vi "Playing.vi"() -> ()   [LabVIEW 2015]
uses:
  SubVIs/Module.Input.ctl
  SubVIs/Loop.Type.ctl
  SubVIs/Module.Type.ctl
  SubVIs/Input.Type.ctl
  SubVIs/Module.Output.ctl
  SubVIs/Output.Type.ctl
  Classes/Loop/Block Diagram/Block Diagram.lvclass
panel:
  out "error out":errorcluster
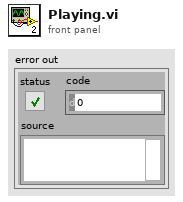
[diagram p1: front panel]
types:
  T1 = cluster{"Name":string, "Type":enum16{"DebugDMA", "Directional Memory", "Analog Replay Memory", "Pattern Generation Memory"}}
  T2 = typedef "Module.Input.ctl" = cluster{"Owning.Loop":T3, "Mod.Type":T4, "Mod.Name":string, "Channels":cluster{"IO Name":string, "Signal Name":string, "Type":T5}[]}
  T3 = typedef "Loop.Type.ctl" = enum16{"HighSpeedDigital", "LowSpeedSigital", "AnalogOutput", "AnalogInput"}
  T4 = typedef "Module.Type.ctl" = enum16{"Digital.8 Channels", "Digital.32 Channels", "Analog.16 Channels.FXP24.5"}
  T5 = typedef "Input.Type.ctl" = enum16{"Digital PWM Input", "Digital Static Input", "Analog PWM Input", "Digital Direct Input", "Analog Direct Input", "Digital Event"}
  T6 = enum16{"DebugDMA", "Directional Memory", "Analog Replay Memory", "Pattern Generation Memory"}
  T7 = typedef "Module.Output.ctl" = cluster{"Owning.Loop":T3, "Mod.Type":T4, "Mod.Name":string, "Channels":cluster{"IO Name":string, "Signal Name":string, "Type":T8}[]}
  T8 = typedef "Output.Type.ctl" = enum16{"Digital PWM Output", "Digital Static Output", "Analog Sine Output", "Digital Direct", "Analog Direct", "Analog Replay", "Pattern Generation", "Directional", "Analog Knock"}
  T9 = cluster{"Name":string, "Type":enum16{"DebugDMA", "Directional Memory", "Analog Replay Memory", "Pattern Generation Memory"}}[]
  T10 = cluster{"IO Name":string, "Signal Name":string, "Type":T8}[]
  T11 = typedef "Variables.ctl" = cluster{"Loops":cluster{"Digital.HighSpeed":cluster{"Diagram":refnum<vi>, "Tunnel":refnum<vi>}, "Digital.LowSpeed":cluster{"Diagram":refnum<vi>, "Tunnel":refnum<vi>}, "Analog.Output":cluster{"Diagram":refnum<vi>, "Tunnel":refnum<vi>}, "Analog.Input":cluster{"Diagram":refnum<vi>, "Tunnel":refnum<vi>}}, "DMA":refnum<vi>, "Locations":cluster{"Sequence.Init":refnum<vi>}, "Application Directory":path, "Block Diagram":refnum<vi>, "vi.Lib":path}
  T12 = typedef "LVPointTypeDef.ctl" = cluster{"Horizontal":i16, "Vertical":i16}
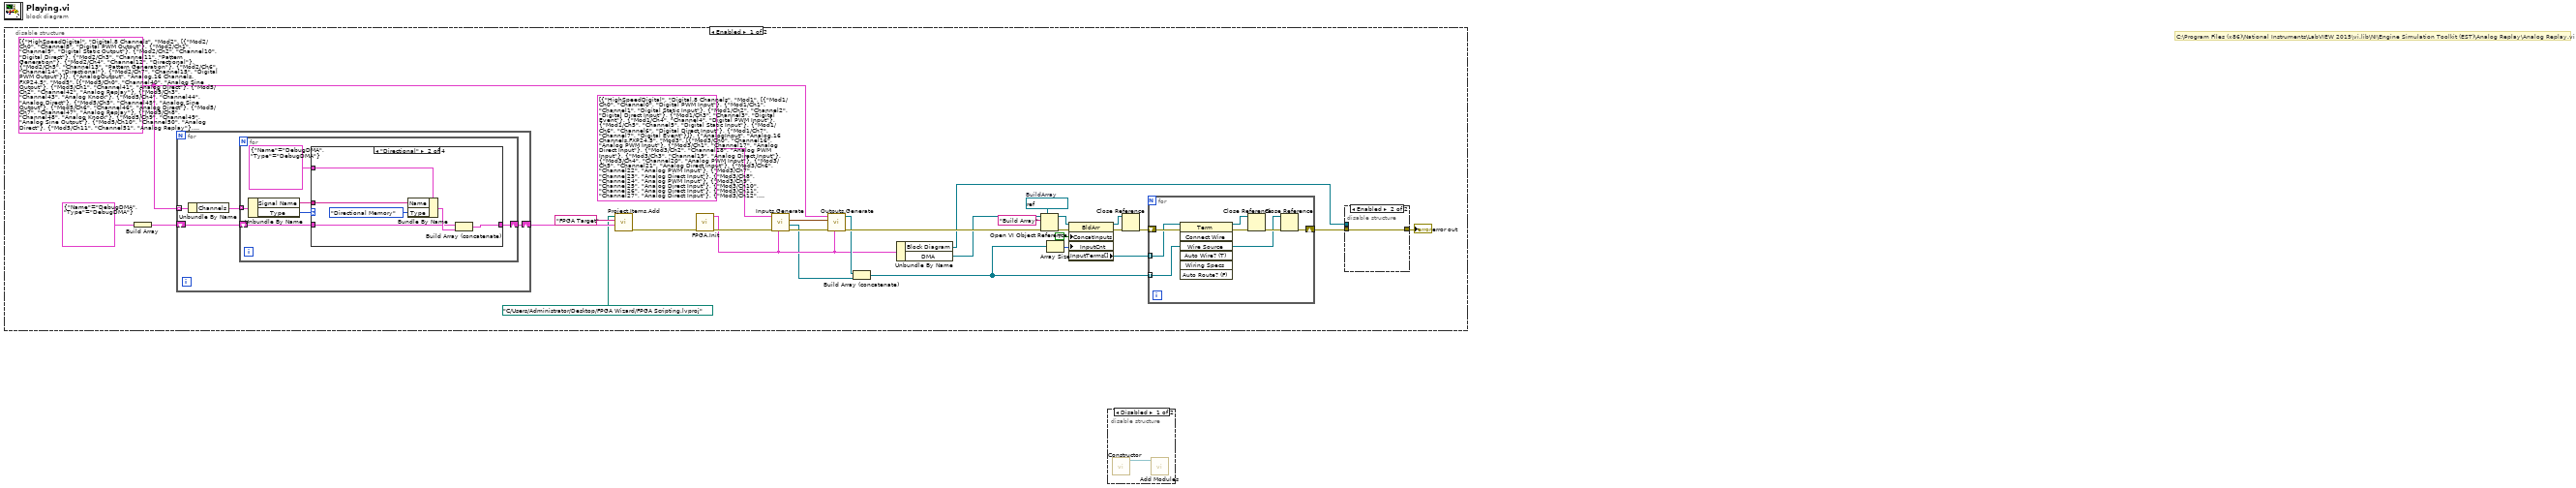
[diagram p0: block diagram]
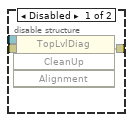
[diagram p3: hidden frame]
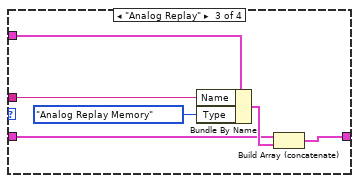
[diagram p5: hidden frame]
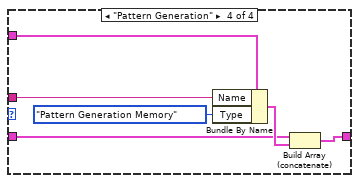
[diagram p6: hidden frame]
diagram:
  # "C:\\Program Files (x86)\\National Instruments\\LabVIEW 2015\\vi.lib\\NI\\Engine Simulation Toolkit (EST)\\Analog Replay\\Analog Replay.vi"
  n1 = disable-structure shown="Enabled" {
    frame Enabled {
      w11 = T7[] [{"Owning.Loop"=enum."HighSpeedDigital", "Mod.Type"=enum."Digital.8 Channels", "Mod.Name"="Mod2", "Channels"=[{"IO Name"="Mod2/Ch0", "Signal Name"="Channel8", "Type"=enum."Digital PWM Output"}, {"IO Name"="Mod2/Ch1", "Signal Name"="Channel9", "Type"=enum."Digital Static Output"}, {"IO Name"="Mod2/Ch2", "Signal Name"="Channel10", "Type"=enum."Digital Direct"}, {"IO Name"="Mod2/Ch3", "Signal Name"="Channel11", "Type"=enum."Pattern Generation"}, {"IO Name"="Mod2/Ch4", "Signal Name"="Channel12", "Type"=enum."Directional"}, {"IO Name"="Mod2/Ch5", "Signal Name"="Channel13", "Type"=enum."Pattern Generation"}, {"IO Name"="Mod2/Ch6", "Signal Name"="Channel14", "Type"=enum."Directional"}, {"IO Name"="Mod2/Ch7", "Signal Name"="Channel15", "Type"=enum."Digital PWM Output"}]}, {"Owning.Loop"=enum."AnalogOutput", "Mod.Type"=enum."Analog.16 Channels.FXP24.5", "Mod.Name"="Mod5", "Channels"=[{"IO Name"="Mod5/Ch0", "Signal Name"="Channel40", "Type"=enum."Analog Sine Output"}, {"IO Name"="Mod5/Ch1", "Signal Name"="Channel41", "Type"=enum."Analog Direct"}, {"IO Name"="Mod5/Ch2", "Signal Name"="Channel42", "Type"=enum."Analog Replay"}, {"IO Name"="Mod5/Ch3", "Signal Name"="Channel43", "Type"=enum."Analog Knock"}, {"IO Name"="Mod5/Ch4", "Signal Name"="Channel44", "Type"=enum."Analog Direct"}, {"IO Name"="Mod5/Ch5", "Signal Name"="Channel45", "Type"=enum."Analog Sine Output"}, {"IO Name"="Mod5/Ch6", "Signal Name"="Channel46", "Type"=enum."Analog Direct"}, {"IO Name"="Mod5/Ch7", "Signal Name"="Channel47", "Type"=enum."Analog Replay"}, {"IO Name"="Mod5/Ch8", "Signal Name"="Channel48", "Type"=enum."Analog Knock"}, {"IO Name"="Mod5/Ch9", "Signal Name"="Channel49", "Type"=enum."Analog Sine Output"}, {"IO Name"="Mod5/Ch10", "Signal Name"="Channel50", "Type"=enum."Analog Direct"}, {"IO Name"="Mod5/Ch11", "Signal Name"="Channel51", "Type"=enum."Analog Replay"}, {"IO Name"="Mod5/Ch12", "Signal Name"="Channel52", "Type"=enum."Analog Knock"}, {"IO Name"="Mod5/Ch13", "Signal Name"="Channel53", "Type"=enum."Analog Replay"}, {"IO Name"="Mod5/Ch14", "Signal Name"="Channel54", "Type"=enum."Analog Direct"}, {"IO Name"="Mod5/Ch15", "Signal Name"="Channel55", "Type"=enum."Analog Sine Output"}]}] ("Outputs")
      w29 = refnum<vi> refnum  # BuildArray
      n2 = Build Array(T1 {"Name"="DebugDMA", "Type"=enum."DebugDMA"}) -> (w9:T9)
      n3 = for {
        tunnel: w11 -> [w45] mode=indexing
        shift-right: [w42] -> w8
        shift-left: w9 -> [w43]
        n4 = Unbundle By Name(w45) -> ("Channels"=w44:T10)
        n5 = for {
          tunnel: w44 -> [w51] mode=indexing
          shift-right: [w46] -> w42
          shift-left: w43 -> [w47]
          n6 = Unbundle By Name(w51) -> ("Signal Name"=w49:string, "Type"=w50:T8)
          n7 = case shown="\"Directional\"" w50 {
            tunnel: w49 -> [_ w57 w63 w69]
            tunnel: T1 {"Name"="DebugDMA", "Type"=enum."DebugDMA"} -> [_ w58 w64 w70]
            tunnel: w47 -> [w52 w54 w60 w66]
            tunnel: [w52 w53 w59 w65] -> w46
            frame Default {
            }
            frame "Directional" {
              n8 = Bundle By Name(cluster=w58, "Name"=w57, "Type"=T6."Directional Memory") -> (w55:T1)
              n9 = Build Array (concatenate)(w54, w55) -> (w53:T9)
            }
            frame "Analog Replay" {
              n10 = Bundle By Name(cluster=w64, "Name"=w63, "Type"=T6."Analog Replay Memory") -> (w61:T1)
              n11 = Build Array (concatenate)(w60, w61) -> (w59:T9)
            }
            frame "Pattern Generation" {
              n12 = Bundle By Name(cluster=w70, "Name"=w69, "Type"=T6."Pattern Generation Memory") -> (w67:T1)
              n13 = Build Array (concatenate)(w66, w67) -> (w65:T9)
            }
          }
        }
      }
      n14 = call "Project.Items.Add.vi"("Array"=w8, "FPGA Target Name"="FPGA Target", "Path"=path "C:/Users/Administrator/Desktop/FPGA Wizard/FPGA Scripting.lvproj") -> ("error out"=w18:errorcluster)  [unwired: 8 in]
      n15 = call "FPGA.Init.vi"("error in (no error)"=w18) -> ("error out"=w19:errorcluster, "Cluster"=w5:T11)  [unwired: 9 in]
      n16 = call "Inputs.Generate.vi"("Variables"=w5, "error in (no error)"=w19, "Inputs"=T2[] [{"Owning.Loop"=enum."HighSpeedDigital", "Mod.Type"=enum."Digital.8 Channels", "Mod.Name"="Mod1", "Channels"=[{"IO Name"="Mod1/Ch0", "Signal Name"="Channel0", "Type"=enum."Digital PWM Input"}, {"IO Name"="Mod1/Ch1", "Signal Name"="Channel1", "Type"=enum."Digital Static Input"}, {"IO Name"="Mod1/Ch2", "Signal Name"="Channel2", "Type"=enum."Digital Direct Input"}, {"IO Name"="Mod1/Ch3", "Signal Name"="Channel3", "Type"=enum."Digital Event"}, {"IO Name"="Mod1/Ch4", "Signal Name"="Channel4", "Type"=enum."Digital PWM Input"}, {"IO Name"="Mod1/Ch5", "Signal Name"="Channel5", "Type"=enum."Digital Static Input"}, {"IO Name"="Mod1/Ch6", "Signal Name"="Channel6", "Type"=enum."Digital Direct Input"}, {"IO Name"="Mod1/Ch7", "Signal Name"="Channel7", "Type"=enum."Digital Event"}]}, {"Owning.Loop"=enum."AnalogInput", "Mod.Type"=enum."Analog.16 Channels.FXP24.5", "Mod.Name"="Mod3", "Channels"=[{"IO Name"="Mod3/Ch0", "Signal Name"="Channel16", "Type"=enum."Analog PWM Input"}, {"IO Name"="Mod3/Ch1", "Signal Name"="Channel17", "Type"=enum."Analog Direct Input"}, {"IO Name"="Mod3/Ch2", "Signal Name"="Channel18", "Type"=enum."Analog PWM Input"}, {"IO Name"="Mod3/Ch3", "Signal Name"="Channel19", "Type"=enum."Analog Direct Input"}, {"IO Name"="Mod3/Ch4", "Signal Name"="Channel20", "Type"=enum."Analog PWM Input"}, {"IO Name"="Mod3/Ch5", "Signal Name"="Channel21", "Type"=enum."Analog Direct Input"}, {"IO Name"="Mod3/Ch6", "Signal Name"="Channel22", "Type"=enum."Analog PWM Input"}, {"IO Name"="Mod3/Ch7", "Signal Name"="Channel23", "Type"=enum."Analog Direct Input"}, {"IO Name"="Mod3/Ch8", "Signal Name"="Channel24", "Type"=enum."Analog PWM Input"}, {"IO Name"="Mod3/Ch9", "Signal Name"="Channel25", "Type"=enum."Analog Direct Input"}, {"IO Name"="Mod3/Ch10", "Signal Name"="Channel26", "Type"=enum."Analog Direct Input"}, {"IO Name"="Mod3/Ch11", "Signal Name"="Channel27", "Type"=enum."Analog Direct Input"}, {"IO Name"="Mod3/Ch12", "Signal Name"="Channel28", "Type"=enum."Analog Direct Input"}, {"IO Name"="Mod3/Ch13", "Signal Name"="Channel29", "Type"=enum."Analog Direct Input"}, {"IO Name"="Mod3/Ch14", "Signal Name"="Channel30", "Type"=enum."Analog Direct Input"}, {"IO Name"="Mod3/Ch15", "Signal Name"="Channel31", "Type"=enum."Analog PWM Input"}]}, {"Owning.Loop"=enum."HighSpeedDigital", "Mod.Type"=enum."Digital.8 Channels", "Mod.Name"="Mod4", "Channels"=[{"IO Name"="Mod4/Ch0", "Signal Name"="Channel32", "Type"=enum."Digital PWM Input"}, {"IO Name"="Mod4/Ch1", "Signal Name"="Channel33", "Type"=enum."Digital Static Input"}, {"IO Name"="Mod4/Ch2", "Signal Name"="Channel34", "Type"=enum."Digital Direct Input"}, {"IO Name"="Mod4/Ch3", "Signal Name"="Channel35", "Type"=enum."Digital Event"}, {"IO Name"="Mod4/Ch4", "Signal Name"="Channel36", "Type"=enum."Digital PWM Input"}, {"IO Name"="Mod4/Ch5", "Signal Name"="Channel37", "Type"=enum."Digital Static Input"}, {"IO Name"="Mod4/Ch6", "Signal Name"="Channel38", "Type"=enum."Digital Direct Input"}, {"IO Name"="Mod4/Ch7", "Signal Name"="Channel39", "Type"=enum."Digital Event"}]}]) -> ("error out"=w16:errorcluster, "Locals.Ref"=w2:refnum<vi>[], "Loop Locations"=w1:T12[])  [unwired: 6 in]
      n17 = call "Outputs.Generate.vi"("Cluster"=w5, "error in (no error)"=w16, "Loop Locations"=w1, "Outputs"=w11) -> ("error out"=w15:errorcluster, "Locals.Ref"=w14:refnum<vi>[])  [unwired: 6 in]
      n18 = Build Array (concatenate)(w14, w2) -> (w13:refnum<vi>[])
      n19 = Unbundle By Name(w5) -> ("Block Diagram"=w3:refnum<vi>, "DMA"=w4:refnum<vi>)
      n20 = Open VI Object Reference(7:w29, 8:w15, 10:"Build Array" ("name/order"), 11:w4) -> (0:w27:errorcluster, 3:w28:refnum<vi>)
      n21 = Array Size(array=w13) -> (size(s)=w24:i32)
      n22 = property class="BldArr"(reference=w28, error in=w27, "ConcatInputs"=TRUE ("Concatenate Inputs"), "InputCnt"=w24) -> (reference out=w20:refnum<vi>, error out=w22:errorcluster, "InputTerms[]"=w26:refnum<vi>[])
      n23 = Close Reference(reference=w20, error in (no error)=w22) -> (error out=w21:errorcluster)
      n24 = for {
        tunnel: w26 -> [w40] mode=indexing
        tunnel: w13 -> [w37] mode=indexing
        shift-right: [w35] -> w25
        shift-left: w21 -> [w41]
        n25 = invoke class="Term" method="Connect Wire"(reference=w40, error in=w41, "Wire Source"=w37) -> (reference out=w38:refnum<vi>, error out=w36:errorcluster)  [unwired: 4 in, 5 out]
        n26 = Close Reference(reference=w38, error in (no error)=w36) -> (error out=w39:errorcluster)
        n27 = Close Reference(reference=w37, error in (no error)=w39) -> (error out=w35:errorcluster)
      }
      n28 = disable-structure shown="Enabled" {
        disable-tunnel: w3 -> [w33 _]
        disable-tunnel: [w32 w34] -> w17
        disable-tunnel: w25 -> [w31 w34]
        frame Disabled {
          n29 = invoke class="TopLvlDiag" method="CleanUp"(reference=w33, error in=w31) -> (error out=w32:errorcluster)  [unwired: 2 in, 3 out]
        }
        frame Enabled {
        }
      }
      "error out" <- w17
    }
    frame Disabled {
    }
  }
  n30 = disable-structure shown="Disabled" {
    frame Disabled {
      n31 = call "Constructor.vi"() -> ("Block Diagram"=w71:refnum<class "Block Diagram.lvclass">)  [unwired: 10 in, 1 out]
      n32 = call "Add Modules.vi"("Block Diagram in"=w71) -> ()  [unwired: 9 in, 2 out]
    }
    frame Enabled {
    }
  }
